vi "K_S30_VISA F95.vi"(4 "error in":errorcluster, 5 "Target Value":sgl format="%.6e", 6 "Command":T1(ring), 7 "Address":u8=250) -> (0 "error out":errorcluster)   [LabVIEW 2012]
panel:
  # "Function 95: Zero\nV1.0, b.v."
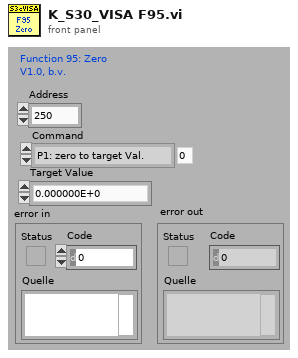
[diagram p1: front panel]
types:
  T1 = enum8{"P1: zero to target Val.", "P1: reset zero", "P2: zero to target Val.", "P2: reset zero", "cmd 4", "cmd 5", "CH0: zero to target Val.", "CH0: reset zero"}
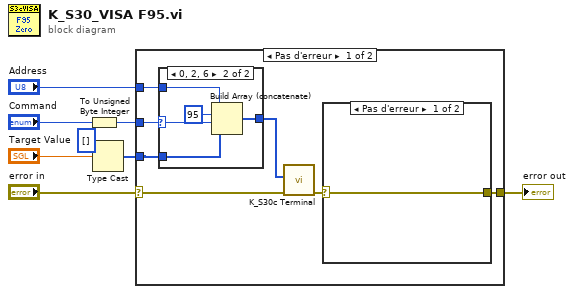
[diagram p0: block diagram]
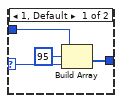
[diagram p2: hidden frame]
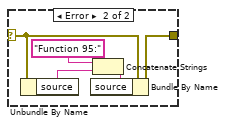
[diagram p3: hidden frame]
diagram:
  n1 = To Unsigned Byte Integer(number="Command") -> (unsigned 8bit integer=w1:u8)
  n2 = Type Cast(type=u8[] [] ("response"), x="Target Value") -> (*(type *) &x=w3:u8[])
  n3 = case shown="Pas d'erreur" "error in" {
    selector: "error in" -> [w13 w31]
    tunnel: "Address" -> [w15 _]
    tunnel: [w11 w31] -> w6
    tunnel: w3 -> [w9 _]
    tunnel: w1 -> [w10 _]
    frame No Error {
      n4 = case shown="0, 2, 6" w10 {
        selector: w10 -> [w16 w21]
        tunnel: w15 -> [w19 w24]
        tunnel: [w17 w22] -> w14
        tunnel: w9 -> [_ w20]
        frame 1, Default {
          n5 = Build Array(w19, u8 95 ("Element"), w16) -> (w17:u8[])
        }
        frame 0, 2, 6 {
          n6 = Build Array (concatenate)(w24, u8 95 ("Element"), w21, w20) -> (w22:u8[])
        }
      }
      n7 = call "K_S30c Terminal.vi"("error in"=w13, "request"=w14) -> ("error out"=w12:errorcluster)  [unwired: 4 in, 1 out]
      n8 = case shown="Pas d'erreur" w12 {
        selector: w12 -> [w25 w30]
        tunnel: [w25 w28] -> w11
        frame No Error {
        }
        frame Error {
          n9 = Unbundle By Name(w30) -> ("source"=w27:string)
          n10 = Concatenate Strings("Function 95:" ("String"), w27) -> (w29:string)
          n11 = Bundle By Name(cluster=w30, "source"=w29) -> (w28:errorcluster)
        }
      }
    }
    frame Error {
    }
  }
  "error out" <- w6
